vi "LJUD_eAIN.vi"(0 "Handle In":i32, 1 "Range":i32, 2 "Resolution":i32, 3 "Settling":i32, 5 "ChannelP":i32, 7 "ChannelN":i32=199, 11 "error in":errorcluster, 12 "Binary":i32) -> (4 "Handle Out":i32, 6 "Voltage":dbl format="%.6f", 15 "error out":errorcluster)   [LabVIEW 2021]
doc: "This is an easy function to read\na single analog input. On the U3\nthis function also configures the line\nas analog if needed.\n\nSee Sections 4.2 and 4.3 of the device's\ndatasheet for more information.\n\nRange: \nU3 - N/A\nU6 - LJ_rgBIP10V=+/-10V, LJ_rgBIP1V=+/- 1V, LJ_rgBIPP1V=+/- 0.1V, LJ_rgBIPP01V=+/-0.01V\nUE9 - LJ_rgUNI5V=0-5V, LJ_rgUNI2P5V=0-2.5V, LJ_rgUNI1P25V=0-1.25V, LJ_rgUNIP625V=0-0.625V, LJ_rgBIP5V=+/- 5V\n\nResolution:\nU3 - QuickSample if TRUE\nU6 - 0=default, 1-8=high-speed ADC, 9-12=high-res ADC\nUE9 - 0=default, 1-17=normal ADC, 18=high-res ADC\n\nSettling:\nU3 - LongSettling if TRUE\nU6 - 0-9 where 0=Auto, see Section 5.2.5.2"
uses:
  labjackud.dll
panel:
  # "This is an easy function to read\na single analog input.  On the U3\nthis function also configures the line\nas analog if needed.\n\nSee Sections 4.2 and 4.3 of the device's\ndatasheet for more information.\n\nRange:  \nU3 - N/A\nU6 - LJ_rgBIP10V=+/-10V, LJ_rgBIP1V=+/- 1V, LJ_rgBIPP1V=+/- 0.1V, LJ_rgBIPP01V=+/-0.01V\nUE9 - LJ_rgUNI5V=0-5V, LJ_rgUNI2P5V=0-2.5V, LJ_rgUNI1P25V=0-1.25V, LJ_rgUNIP625V=0-0.625V, LJ_rgBIP5V=+/- 5V\n\nResolution:\nU3 - QuickSample if TRUE\nU6 - 0=default, 1-8=high-speed ADC, 9-12=high-res ADC\nUE9 - 0=default, 1-17=normal ADC, 18=high-res ADC\n\nSettling:\nU3 - LongSettling if TRUE\nU6 - 0-9 where 0=Auto, see Section 5.2.5.2"
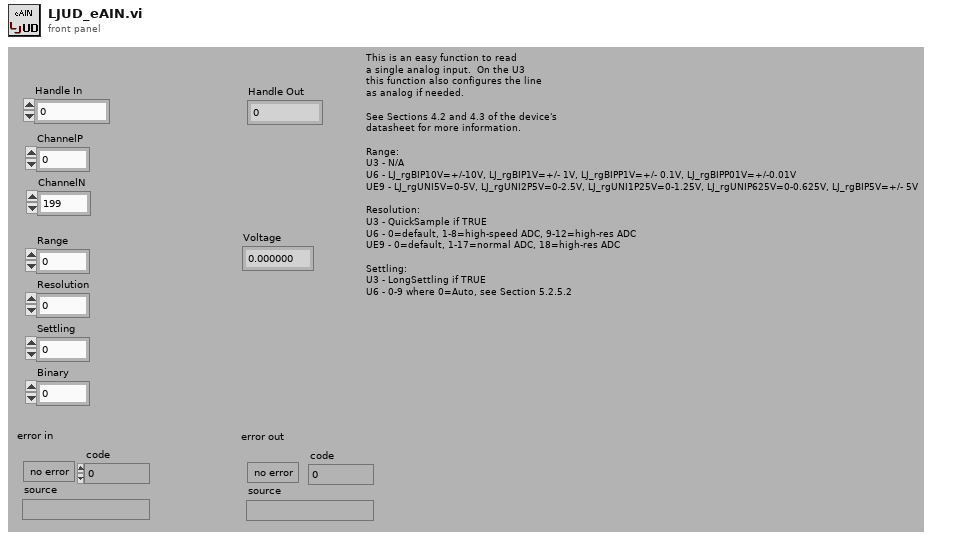
[diagram p1: front panel]
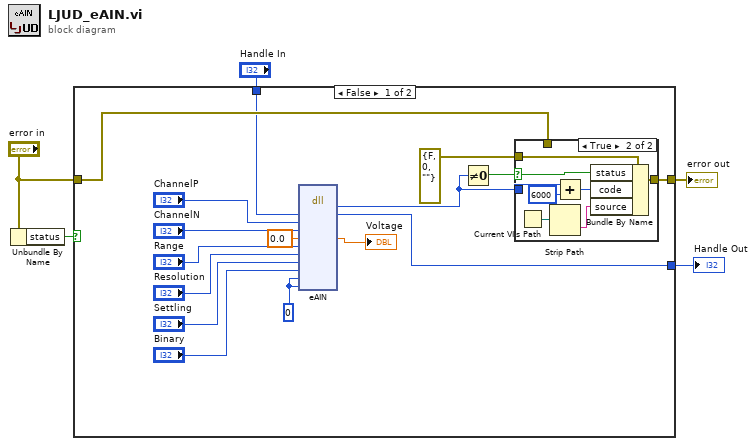
[diagram p0: block diagram]
diagram:
  n1 = Unbundle By Name("error in") -> ("status"=w4:bool)
  n2 = case shown="False" w4 {
    tunnel: [w18 w32] -> w5
    tunnel: "error in" -> [w17 w32]
    tunnel: "Handle In" -> [w7 w31]
    tunnel: [w6 w31] -> w1
    frame False {
      w8 = 0 ("Reserved1")
      n3 = dll-call lib="labjackud.dll" fn="eAIN"("Handle"=w7, "ChannelP"="ChannelP", "ChannelN"="ChannelN", "Voltage"=0.0, "Range"="Range", "Resolution"="Resolution", "Settling"="Settling", "Binary"="Binary", "Reserved1"=w8, "Reserved2"=w8) -> (w19:i32, "Handle"=w6:i32, "Voltage"=→"Voltage":dbl)  [unwired: 11 in, 2 out]
      n4 = Not Equal To 0?(x=w19) -> (x != 0?=w20:bool)
      n5 = case shown="True" w20 {
        selector: w20 -> [_ w29]
        tunnel: [w22 w30] -> w18
        tunnel: errorcluster {"status"=FALSE, "code"=0, "source"=""} ("error IO") -> [_ w28]
        tunnel: w19 -> [_ w24]
        tunnel: w17 -> [w22 _]
        frame False {
        }
        frame True {
          n6 = Current VI's Path() -> (path=w26:path)
          n7 = Strip Path(path=w26) -> (name=w27:string)  [unwired: 1 out]
          n8 = Add(x=w24, y=6000) -> (x+y=w25:i32)
          n9 = Bundle By Name(cluster=w28, "status"=w29, "code"=w25, "source"=w27) -> (w30:errorcluster)
        }
      }
    }
    frame True {
    }
  }
  "error out" <- w5
  "Handle Out" <- w1
